vi "next state.vi"(8 "error in":errorcluster, 10 "thread queue":refnum<queue>, 11 "state queue in":string[](array[string])) -> (0 "error out":errorcluster, 1 "data":variant, 2 "next state":string, 3 "state queue out":string[](array[string]), 4 "previous state":string)   [LabVIEW 2012]
doc: "Example of implementing an architecture for interactive LabVIEW applications. See the \"Interactive Architectures Revisited\" article in the LabVIEW Technical Resource newsletter, Spring 1996 issue for more details.\n\nSubscribe to the LabVIEW Technical Resource newsletter!\nContact:\nLTR Publishing\n5614 Anita\nDallas, TX 75206\n(214) 827-9931\nFAX (214) 827-9932\nemail ltrsub@aol.com"
uses:
  interthread comms/typedefs/interthread message.ctl
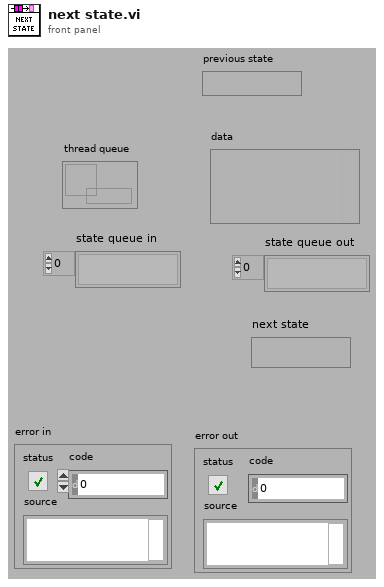
[diagram p1: front panel]
types:
  T1 = typedef "interthread message.ctl" = cluster{"destination state":string, "data":variant}
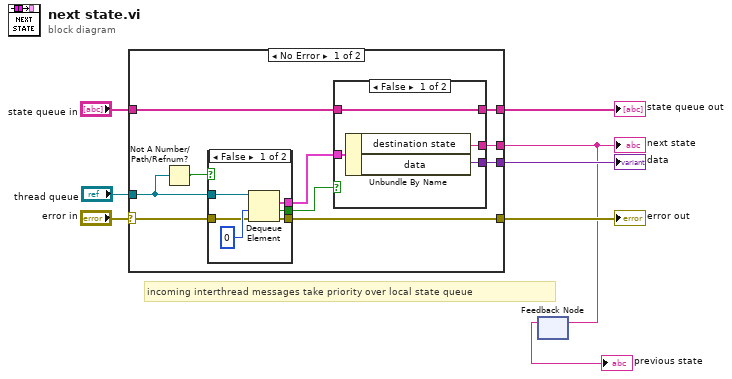
[diagram p0: block diagram]
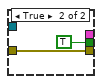
[diagram p2: hidden frame]
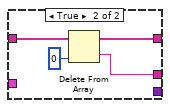
[diagram p3: hidden frame]
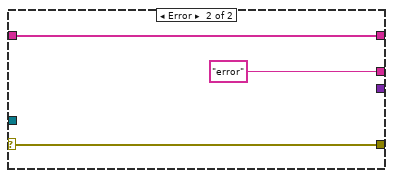
[diagram p4: hidden frame]
diagram:
  # "incoming interthread messages take priority over local state queue"
  n1 = case shown="No Error" "error in" {
    selector: "error in" -> [w15 w37]
    tunnel: "state queue in" -> [w18 w36]
    tunnel: [w17 w36] -> w8
    tunnel: [w16 "error"] -> w2
    tunnel: [w14 w37] -> w7
    tunnel: "thread queue" -> [w10 _]
    tunnel: [w11 _] -> w3
    frame No Error {
      n2 = Not A Number/Path/Refnum?(number/path/refnum=w10) -> (NaN/Path/Refnum?=w9:bool)
      n3 = case shown="False" w9 {
        tunnel: w15 -> [w23 w26]
        tunnel: [w22 w26] -> w14
        tunnel: [w21 TRUE ("timed out?")] -> w13
        tunnel: [w20 _] -> w12
        tunnel: w10 -> [w19 _]
        frame False {
          n4 = Dequeue Element(queue=w19, timeout in ms (-1)=0, error in (no error)=w23) -> (element=w20:T1, timed out?=w21:bool, error out=w22:errorcluster)  [unwired: 1 out]
        }
        frame True {
        }
      }
      n5 = case shown="False" w13 {
        tunnel: w18 -> [w30 w34]
        tunnel: [w30 w33] -> w17
        tunnel: [w28 w32] -> w16
        tunnel: w12 -> [w29 _]
        tunnel: [w27 _] -> w11
        frame False {
          n6 = Unbundle By Name(w29) -> ("destination state"=w28:string, "data"=w27:variant)
        }
        frame True {
          n7 = Delete From Array(array=w34, index=0 ("Index")) -> (deleted portion=w32:string, array with subset deleted=w33:string[])  [unwired: 1 in]
        }
      }
    }
    frame Error {
    }
  }
  "state queue out" <- w8
  "next state" <- w2
  "error out" <- w7
  "data" <- w3
  n8 = feedback-in #1(w2) -> ()
  n9 = feedback #1() -> (→"previous state":string)  [unwired: 1 in]
